vi "Reinitialize.vi"(8 "error in (no error)":errorcluster, 11 "Registry in":refnum<class "Registry.lvclass">) -> (0 "error out":errorcluster, 3 "Registry out":refnum<class "Registry.lvclass">)   [LabVIEW 2020, in "BCI-1553 API.lvlib" / "Registry.lvlib" / "Registry.lvclass"]
doc: "Re-initializes the Registry to be empty."
uses:
  Registry.lvclass
  Registry.lvclass/Registry.ctl
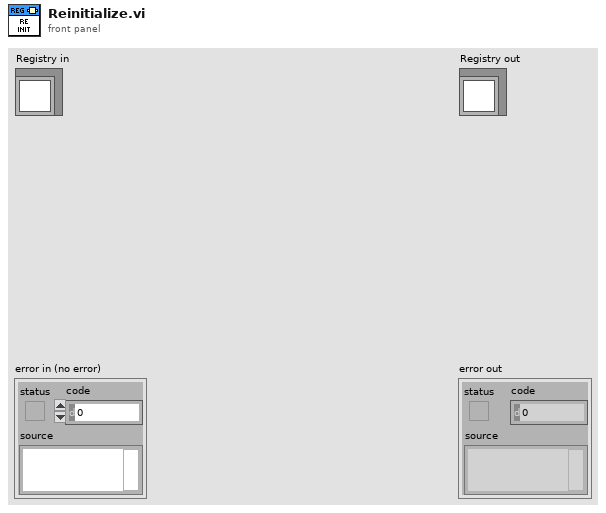
[diagram p1: front panel]
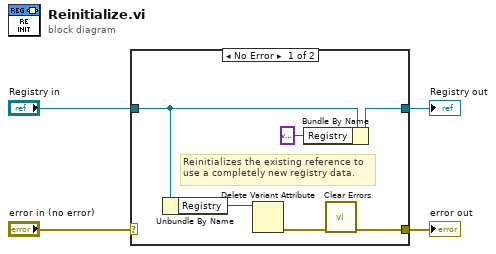
[diagram p0: block diagram]
diagram:
  n1 = case shown="No Error" "error in (no error)" {
    selector: "error in (no error)" -> [_ w12]
    tunnel: [w5 w12] -> w3
    tunnel: [w10 w11] -> w1
    tunnel: "Registry in" -> [w8 w11]
    frame No Error {
      # "Reinitializes the existing reference to\nuse a completely new registry data."
      n2 = Unbundle By Name(w8) -> ("Registry"=w7:variant)
      n3 = Delete Variant Attribute(7:w7) -> (0:w6:errorcluster)  [unwired: 2 in, 2 out]
      n4 = Bundle By Name(cluster=w8, "Registry"=variant) -> (w10:refnum<class "Registry.lvclass">)
      n5 = call <vilib>:"Clear Errors.vi"("error in (no error)"=w6) -> ("error out"=w5:errorcluster)  [unwired: 5 in, 1 out]
    }
    frame Error {
    }
  }
  "error out" <- w3
  "Registry out" <- w1
